vi "Convert Message.vi"(8 "error in (no error)":errorcluster, 11 "Engine RPM in":refnum<class "Fuel Level Input.lvclass">) -> (0 "error out":errorcluster, 1 "variant":variant, 2 "Result":dbl, 3 "Engine RPM out":refnum<class "Fuel Level Input.lvclass">)   [LabVIEW 2011, in "Fuel Level Input.lvclass"]
uses:
  Fuel Level Input.lvclass
  PID.lvclass
panel:
  out "number":u16
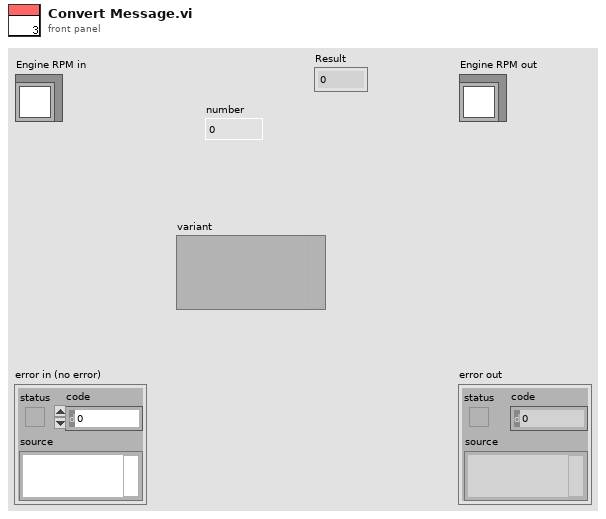
[diagram p1: front panel]
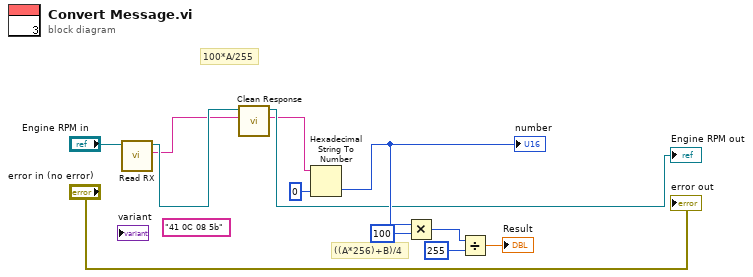
[diagram p0: block diagram]
diagram:
  (unwired) "41 0C 08 5b" ("regular expression")
  # "100*A/255"
  # "((A*256)+B)/4"
  n1 = call "Read RX.vi"("PID in"="Engine RPM in") -> ("RX"=w1:string, "PID out"=w2:refnum<class "Fuel Level Input.lvclass">)  [unwired: 8 in, 1 out]
  n2 = call-dynamic "Clean Response.vi"("Response In"=w1, "PID.lvclass"=w2) -> ("result string"=w4:string, "PID.lvclass 2"=→"Engine RPM out":refnum<class "Fuel Level Input.lvclass">)  [unwired: 7 in, 1 out]
  n3 = Hexadecimal String To Number(string=w4, default (0uL)=u16 0 ("default (0 U32)")) -> (number=w11:u16)  [unwired: 1 in, 1 out]
  "number" <- w11
  n4 = Multiply(x=w11, y=u16 100) -> (x*y=w9:u16)
  n5 = Divide(x=w9, y=u16 255) -> (x/y=→"Result":dbl)
  "error out" <- "error in (no error)"
